vi "Open Connection to Target.vi"(8 "error in (no error)":errorcluster, 10 "IP Address":string, 11 "TCP Service":string) -> (0 "error out":errorcluster, 3 "connection info":T1)   [LabVIEW 2023, in "J1939 Addon Shared.lvlib"]
uses:
  J1939 Addon Shared.lvlib
  <vilib>/NI/STM/TCP/TCP Connection Info.ctl
  <vilib>/NI/STM/SubVIs/MetaDataElement.ctl
  <vilib>/NI/STM/TCP/TCP Write Options.ctl
  <vilib>/NI/STM/TCP/Write Meta Data (TCP Ref).vi
  <vilib>/NI/STM/TCP/Write Meta Data (TCP Clst).vi
  <vilib>/NI/STM/NI STM.lvlib
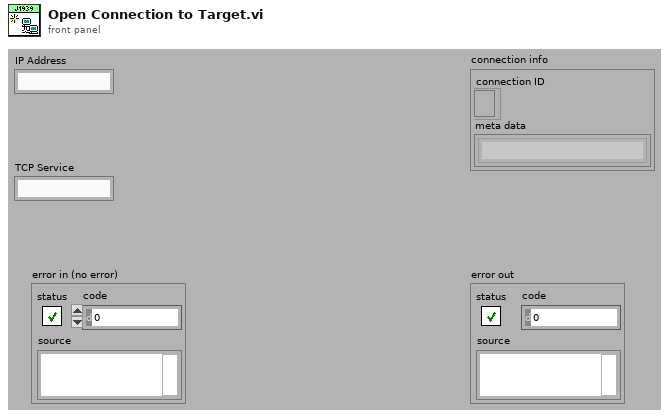
[diagram p1: front panel]
types:
  T1 = typedef "NI STM.lvlib/TCP Connection Info.ctl" = cluster{"connection ID":refnum<k5>, "meta data":T2[]}
  T2 = typedef "NI STM.lvlib/MetaDataElement.ctl" = string
  T3 = typedef "NI STM.lvlib/TCP Write Options.ctl" = cluster{"ignore timeout error":bool, "timeout ms (1000)":i32}
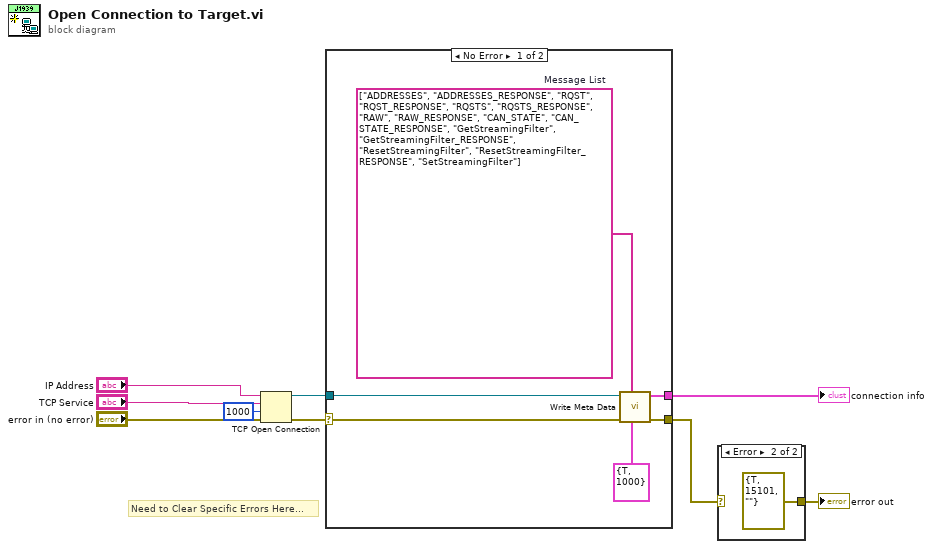
[diagram p0: block diagram]
diagram:
  # "Need to Clear Specific Errors Here..."
  n1 = TCP Open Connection(address="IP Address", remote port or service name="TCP Service", timeout ms (60000)=1000, error in (no error)="error in (no error)") -> (connection ID=w9:refnum<k5>, error out=w8:errorcluster)  [unwired: 1 in]
  n2 = case shown="No Error" w8 {
    selector: w8 -> [w11 w16]
    tunnel: w9 -> [w14 _]
    tunnel: [w13 w16] -> w2
    tunnel: [w12 _] -> w6
    frame No Error {
      w15 = string[] ["ADDRESSES", "ADDRESSES_RESPONSE", "RQST", "RQST_RESPONSE", "RQSTS", "RQSTS_RESPONSE", "RAW", "RAW_RESPONSE", "CAN_STATE", "CAN_STATE_RESPONSE", "GetStreamingFilter", "GetStreamingFilter_RESPONSE", "ResetStreamingFilter", "ResetStreamingFilter_RESPONSE", "SetStreamingFilter"]  # Message List
      n3 = call-poly <vilib>:"Write Meta Data.vi"("options"=T3 {"ignore timeout error"=TRUE, "timeout ms (1000)"=1000}, "meta data"=w15, "error in"=w11, "connection ID"=w14) -> ("error out"=w13:errorcluster, "connection info out"=w12:T1)  [unwired: 6 in]
    }
    frame Error {
    }
  }
  "connection info" <- w6
  n4 = case shown="Error" w2 {
    selector: w2 -> [w17 _]
    tunnel: [w17 errorcluster {"status"=TRUE, "code"=15101, "source"=""} ("error IO")] -> w1
    frame No Error {
    }
    frame Error {
    }
  }
  "error out" <- w1
